vi "reached within accuracy.vi"(8 "error in (no error)":errorcluster, 9 "destination":dbl, 10 "last position sent to stage":dbl, 11 "Autofocus in":refnum<class "Autofocus.lvclass">) -> (0 "error out":errorcluster, 2 "at destination?":bool, 3 "Autofocus out":refnum<class "Autofocus.lvclass">)   [LabVIEW 2012, in "Autofocus.lvclass"]
uses:
  Autofocus.lvclass
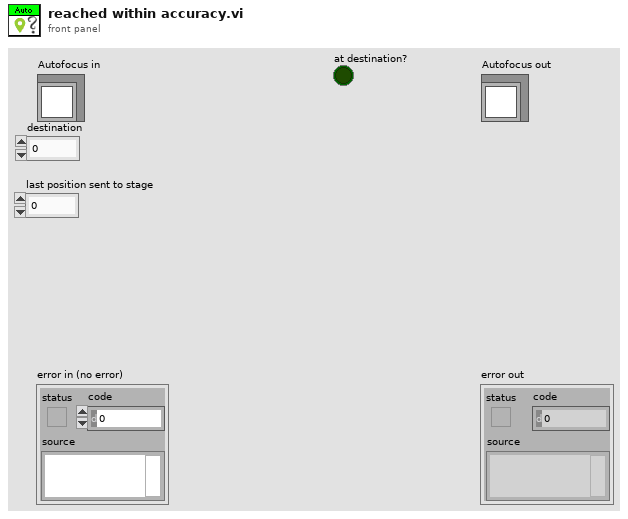
[diagram p1: front panel]
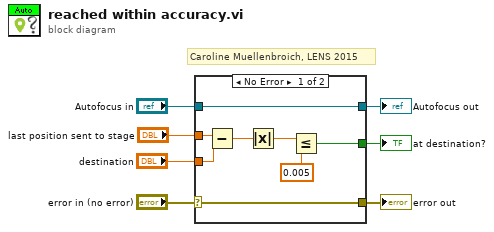
[diagram p0: block diagram]
diagram:
  # "Caroline Muellenbroich, LENS 2015"
  n1 = case shown="No Error" "error in (no error)" {
    selector: "error in (no error)" -> [w14 w17]
    tunnel: [w14 w17] -> w6
    tunnel: [w15 w16] -> w4
    tunnel: "Autofocus in" -> [w15 w16]
    tunnel: "last position sent to stage" -> [w13 _]
    tunnel: "destination" -> [w12 _]
    tunnel: [w8 _] -> w1
    frame No Error {
      n2 = Subtract(x=w13, y=w12) -> (x-y=w11:dbl)
      n3 = Absolute Value(x=w11) -> (abs(x)=w10:dbl)
      n4 = Less Or Equal?(x=w10, y=0.005) -> (x <= y?=w8:bool)
    }
    frame Error {
    }
  }
  "error out" <- w6
  "Autofocus out" <- w4
  "at destination?" <- w1
